vi "Close serial.vi"() -> ()   [LabVIEW 2013]
panel:
  out "error out":errorcluster
  in  "ESP Port":refnum<visa-resource-name>="COM4"
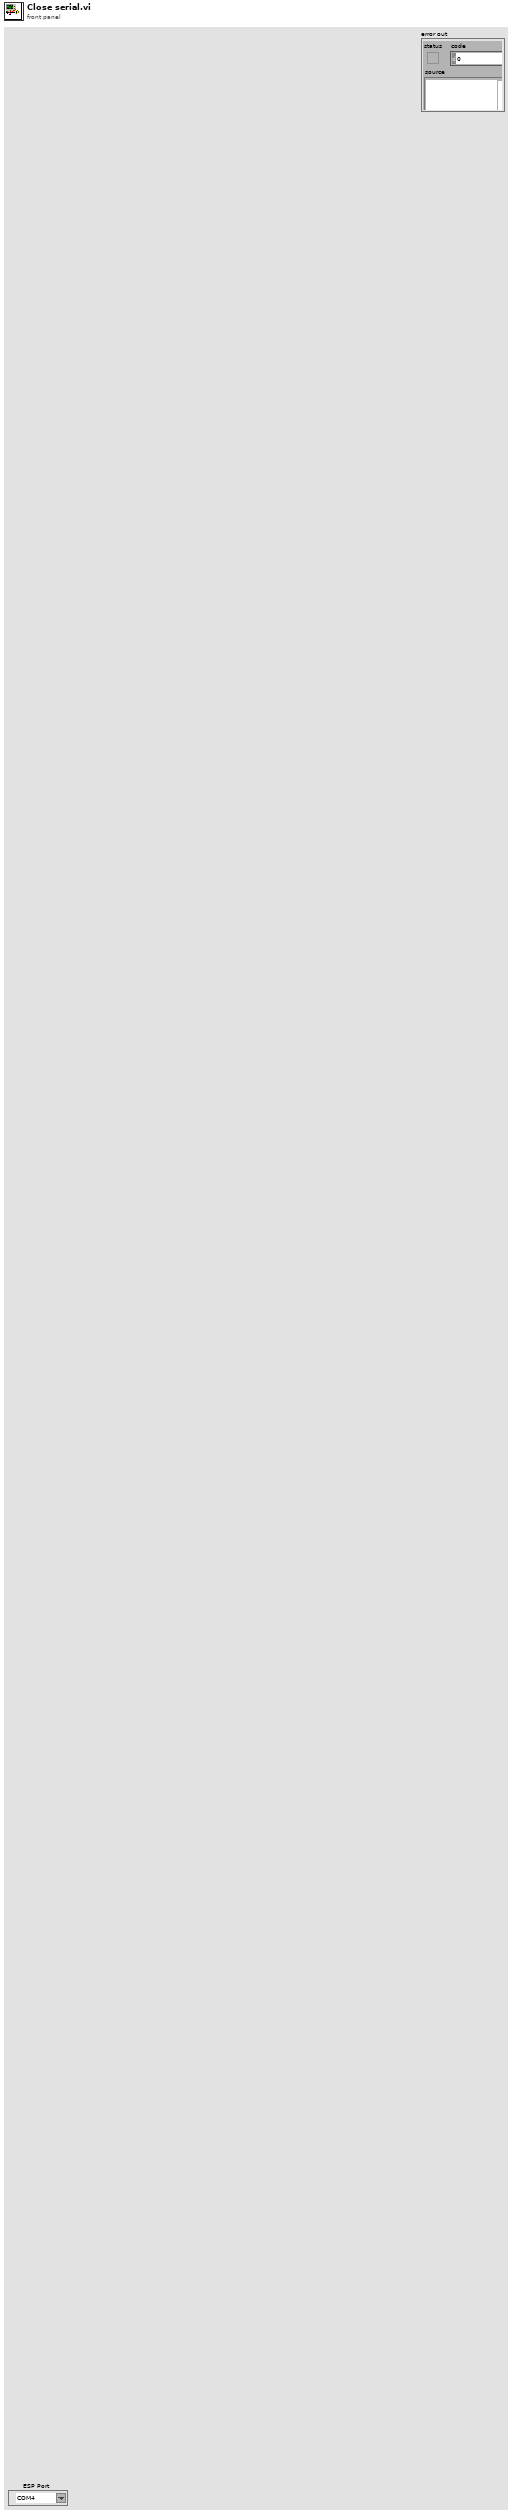
[diagram p1: front panel]
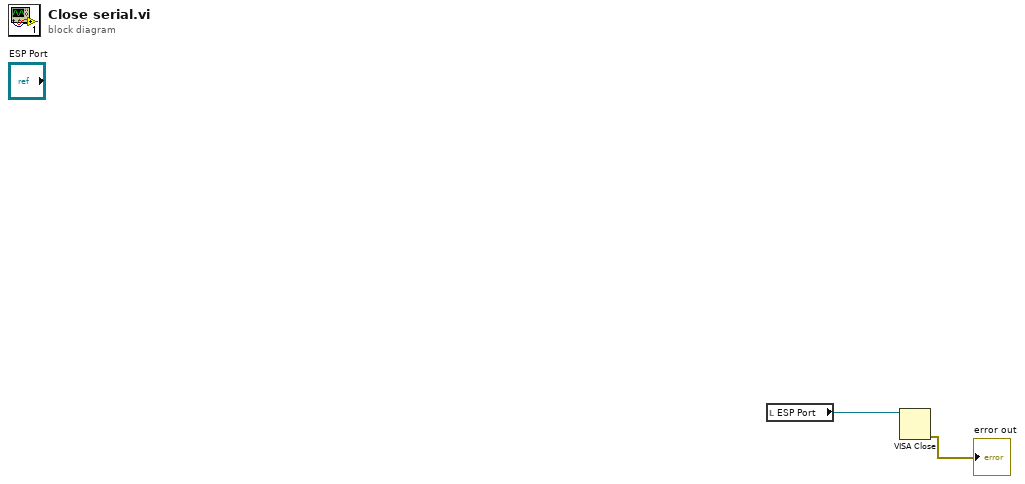
[diagram p0: block diagram]
diagram:
  n1 = local read "ESP Port"() -> (w2:refnum<visa-resource-name>)
  n2 = VISA Close(VISA resource name=w2) -> (error out=→"error out":errorcluster)  [unwired: 1 in]
